vi "Delete elements of variant array.vi"(8 "error in (no error)":errorcluster, 10 "Element to be deleted":u32, 11 "JSON in":variant) -> (0 "error out":errorcluster, 3 "Output JSON":variant)   [LabVIEW 2015]
uses:
  <vilib>/Utility/Data Type/Type Definitions/Data Type.ctl
  <vilib>/Utility/Data Type/NI_Data Type.lvlib
panel:
  out "element":variant
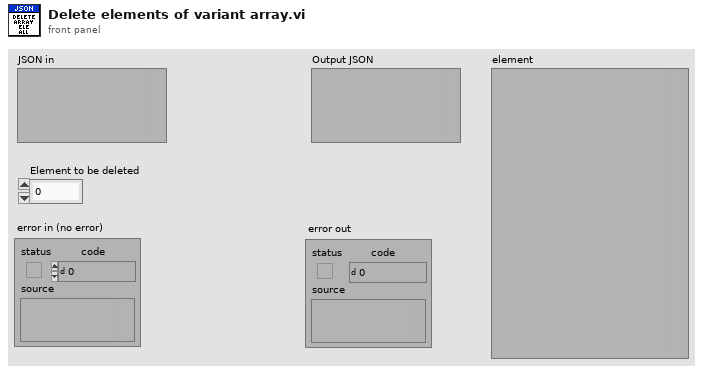
[diagram p1: front panel]
types:
  T1 = typedef "NI_Data Type.lvlib/Data Type.ctl" = enum8{"Invalid Type", "Void", "I8", "I16", "I32", "I64", "U8", "U16", "U32", "U64", "Single Float", "Double Float", "Extended Float", "Single Complex", "Double Complex", "Extended Complex", "Enum U8", "Enum U16", "Enum U32", "Enum U64", "Single Float With Unit", "Double Float With Unit", "Extended Float With Unit", "Single Complex with Unit", "Double Complex with Unit", "Extended Complex with Unit", "Boolean", "String", "Path", "Picture", "Tag", "Array", "Cluster", "Variant", "LV Variant", "Waveform", "Timestamp", "Digital Waveform", "Digital Data", "ExpressData", "Refnum", "External Data", "VI", "Poly VI", "LabVIEW Class Instance", "Fixed Point"}
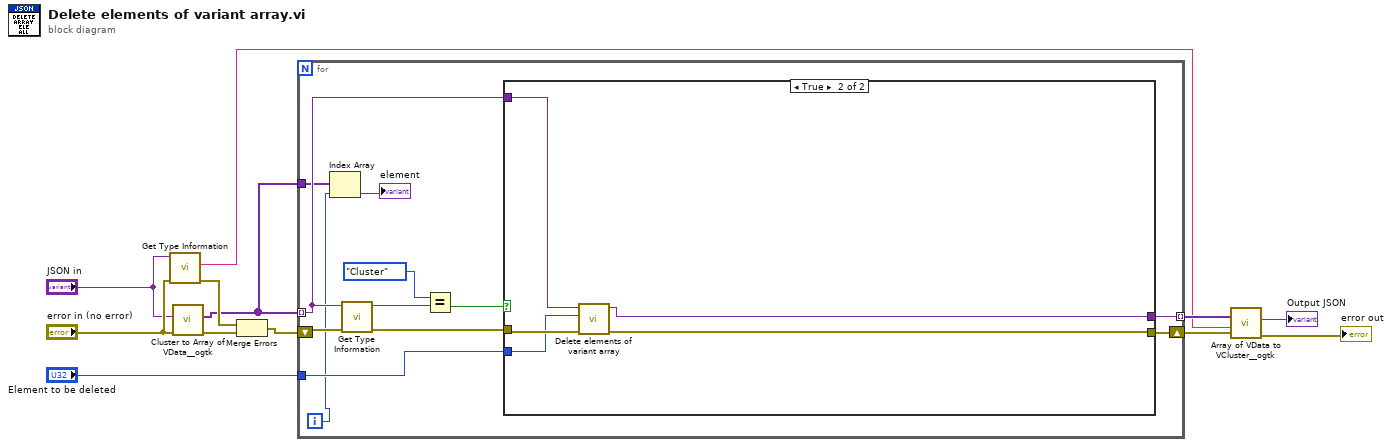
[diagram p0: block diagram]
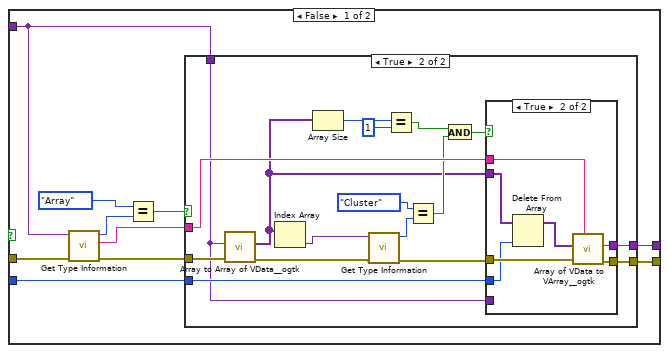
[diagram p2: hidden frame]
diagram:
  n1 = call <vilib>:"Get Type Information.vi"("error in (no error)"="error in (no error)", "Variant"="JSON in") -> ("error out"=w7:errorcluster, "Name"=w6:string)  [unwired: 5 in, 3 out]
  n2 = call <userlib>:"Cluster to Array of VData__ogtk.vi"("error in (no error)"="error in (no error)", "Cluster"="JSON in") -> ("error out"=w5:errorcluster, "Array of VData"=w1:variant[])  [unwired: 8 in]
  n3 = Merge Errors(w7, w5) -> (w3:errorcluster)
  n4 = for {
    tunnel: w1 -> [w19] mode=indexing
    tunnel: "Element to be deleted" -> [w18]
    tunnel: [w17] -> w11 mode=indexing
    shift-right: [w16] -> w10
    shift-left: w3 -> [w24]
    tunnel: w1 -> [w15]
    i -> [w14]
    n5 = Index Array(array=w15, index=w14) -> (element=→"element":variant)
    n6 = call <vilib>:"Get Type Information.vi"("error in (no error)"=w24, "Variant"=w19) -> ("error out"=w23:errorcluster, "Type"=w21:T1)  [unwired: 5 in, 3 out]
    n7 = Equal?(x=Data_Type."Cluster", y=w21) -> (x = y?=w22:bool)
    n8 = case shown="True" w22 {
      tunnel: w23 -> [w34 w67]
      tunnel: w19 -> [w25 w66]
      tunnel: w18 -> [w28 w65]
      tunnel: [w27 w63] -> w16
      tunnel: [w26 w64] -> w17
      frame False {
        n9 = call <vilib>:"Get Type Information.vi"("error in (no error)"=w34, "Variant"=w25) -> ("error out"=w31:errorcluster, "Name"=w30:string, "Type"=w32:T1)  [unwired: 5 in, 2 out]
        n10 = Equal?(x=Data_Type."Array", y=w32) -> (x = y?=w29:bool)
        n11 = case shown="True" w29 {
          tunnel: w25 -> [w35 w37]
          tunnel: w31 -> [w36 w53]
          tunnel: [w35 w52] -> w26
          tunnel: [w36 w51] -> w27
          tunnel: w30 -> [_ w50]
          tunnel: w28 -> [_ w45]
          frame False {
          }
          frame True {
            n12 = call <userlib>:"Array to Array of VData__ogtk.vi"("error in (no error)"=w53, "MultiD Array"=w37) -> ("error out"=w47:errorcluster, "1D Array of Variants"=w38:variant[])  [unwired: 8 in]
            n13 = Index Array(array=w38) -> (element=w44:variant)  [unwired: 1 in]
            n14 = Array Size(array=w38) -> (size(s)=w43:i32)
            n15 = call <vilib>:"Get Type Information.vi"("error in (no error)"=w47, "Variant"=w44) -> ("error out"=w46:errorcluster, "Type"=w48:T1)  [unwired: 5 in, 3 out]
            n16 = Equal?(x=w43, y=1) -> (x = y?=w41:bool)
            n17 = Equal?(x=Data_Type."Cluster", y=w48) -> (x = y?=w40:bool)
            n18 = And(x=w41, y=w40) -> (x .and. y?=w39:bool)
            n19 = case shown="True" w39 {
              tunnel: w46 -> [w55 w62]
              tunnel: [w54 w60] -> w52
              tunnel: [w55 w59] -> w51
              tunnel: w50 -> [_ w58]
              tunnel: w38 -> [_ w57]
              tunnel: w45 -> [_ w56]
              tunnel: w37 -> [w54 _]
              frame False {
              }
              frame True {
                n20 = Delete From Array(array=w57, index=w56) -> (array with subset deleted=w61:variant[])  [unwired: 1 in, 1 out]
                n21 = call <userlib>:"Array of VData to VArray__ogtk.vi"("Array Name"=w58, "error in (no error)"=w62, "1D Array of VData"=w61) -> ("error out"=w59:errorcluster, "VArray"=w60:variant)  [unwired: 7 in]
              }
            }
          }
        }
      }
      frame True {
        n22 = call "Delete elements of variant array.vi"("error in (no error)"=w67, "Element to be deleted"=w65, "JSON in"=w66) -> ("error out"=w63:errorcluster, "Output JSON"=w64:variant)  [unwired: 7 in]
      }
    }
  }
  n23 = call <userlib>:"Array of VData to VCluster__ogtk.vi"("error in (no error)"=w10, "Cluster Name"=w6, "Array"=w11) -> ("error out"=→"error out":errorcluster, "VCluster"=→"Output JSON":variant)  [unwired: 7 in]
